vi "Test Selector.vi"() -> ()   [LabVIEW 2021]
panel:
  out "Array":string[](array[string])
  in  "Test Description":cluster{"Selector":bool, "Test Name":string}[](array[cluster])
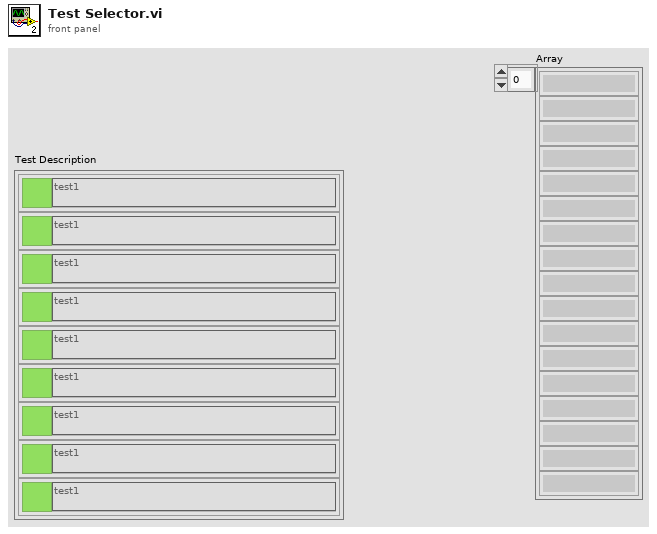
[diagram p1: front panel]
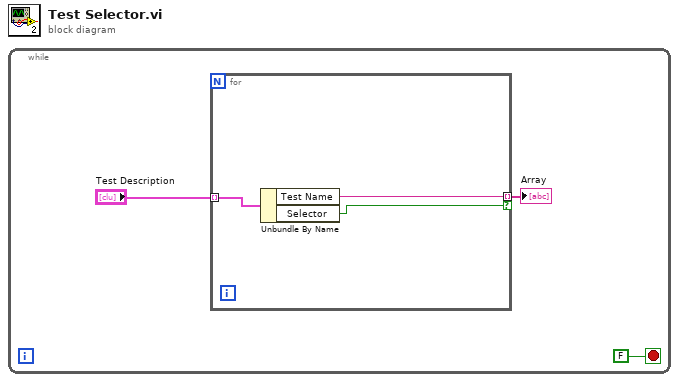
[diagram p0: block diagram]
diagram:
  n1 = while {
    stop <- FALSE stop-if-true
    n2 = for {
      tunnel: "Test Description" -> [w6] mode=indexing
      tunnel: [w5] -> w1 mode=indexing if=w4
      n3 = Unbundle By Name(w6) -> ("Test Name"=w5:string, "Selector"=w4:bool)
    }
    "Array" <- w1
  }
